vi "Tektronix AFG 1000 Series Frequency Sweep.vi"() -> ()   [LabVIEW 2016]
doc: "Demonstrates how to configure and enable a frequency sweep."
uses:
  <instrlib>/Tektronix AFG 1000 Series/Tektronix AFG 1000 Series.lvlib
panel:
  in  "Channel (1 Channel 1)":u16(ring)=1 items=["Channel 1"=1, "Channel 2"=2]
  in  "Enable Frequency Sweep (T: Enable)":bool=TRUE
  in  "Start Frequency (100 Hz)":dbl=100.0 format="%#.6g"
  in  "Stop  Frequency  (1000 Hz)":dbl=1000.0 format="%#.6g"
  in  "Amplitude (1 Vpp)":dbl=1.0
  in  "DC Offset (0.00 V)":dbl
  in  "Waveform Function (0: Sine)":u16(ring) items=["Sine", "Square", "Pulse", "Ramp", "Noise"]
  in  "VISA resource name":refnum<visa-resource-name>
  # "(c) 2016 National Instruments.  ALL RIGHTS RESERVED."
  # "The Pulse, Noise, and DC waveform functions are not valid for Frequency Sweep."
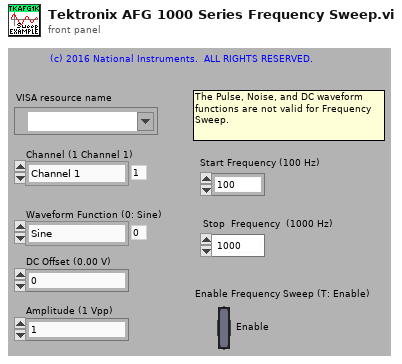
[diagram p1: front panel]
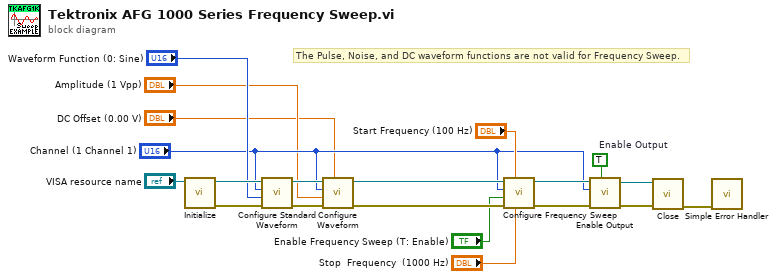
[diagram p0: block diagram]
diagram:
  w10 = TRUE  # Enable Output
  # "The Pulse, Noise, and DC waveform functions are not valid for Frequency Sweep."
  n1 = call <instrlib>:"Initialize.vi"("VISA resource name"="VISA resource name") -> ("error out"=w7:errorcluster, "VISA resource name out"=w6:refnum<visa-resource-name>)  [unwired: 9 in]
  n2 = call <instrlib>:"Configure Standard Waveform.vi"("error in (no error)"=w7, "Waveform Function (0: Sine)"="Waveform Function (0: Sine)", "Channel (1 Channel 1)"="Channel (1 Channel 1)", "VISA resource name"=w6) -> ("error out"=w9:errorcluster, "VISA resource name out"=w8:refnum<visa-resource-name>)  [unwired: 6 in]
  n3 = call <instrlib>:"Configure Waveform.vi"("DC Offset (0.00 V)"="DC Offset (0.00 V)", "error in (no error)"=w9, "Amplitude (1 Vpp)"="Amplitude (1 Vpp)", "Channel (1 Channel 1)"="Channel (1 Channel 1)", "VISA resource name"=w8) -> ("error out"=w19:errorcluster, "VISA resource name out"=w18:refnum<visa-resource-name>)  [unwired: 5 in]
  n4 = call <instrlib>:"Configure Frequency Sweep.vi"("Stop  Frequency  (1000 Hz)"="Stop  Frequency  (1000 Hz)", "Start Frequency (100 Hz)"="Start Frequency (100 Hz)", "error in (no error)"=w19, "Enable Frequency Sweep (T: Enable)"="Enable Frequency Sweep (T: Enable)", "Channel (1: Channel 1)"="Channel (1 Channel 1)", "VISA resource name"=w18) -> ("error out"=w13:errorcluster, "VISA resource name out"=w14:refnum<visa-resource-name>)  [unwired: 4 in]
  n5 = call <instrlib>:"Enable Output.vi"("Enable Output (T: Enable)"=w10, "error in (no error)"=w13, "Channel (1: Channel 1)"="Channel (1 Channel 1)", "VISA resource name"=w14) -> ("error out"=w17:errorcluster, "VISA resource name out"=w16:refnum<visa-resource-name>)  [unwired: 6 in]
  n6 = call <instrlib>:"Close.vi"("error in (no error)"=w17, "VISA resource name"=w16) -> ("error out"=w20:errorcluster)  [unwired: 9 in]
  n7 = call <vilib>:"Simple Error Handler.vi"("error in (no error)"=w20) -> ()  [unwired: 4 in, 5 out]
